vi "AODO-Configure AO.vi"(0 "AO.Channels":string[](array[string]), 5 "AO.Fs (Hz)":dbl, 7 "AO.Npts":i32, 11 "error in (no error)":errorcluster) -> (15 "error out":errorcluster)   [LabVIEW 2020]
uses:
  Typedefs/AODO-Action.ctl
  Typedefs/AODO-Config.ctl
  Typedefs/AODO-Output Spec.ctl
  Typedefs/DO-Output Spec.ctl
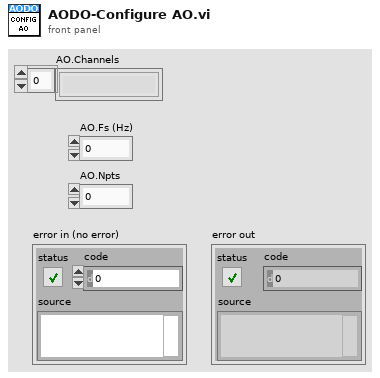
[diagram p1: front panel]
types:
  T1 = typedef "AODO-Config.ctl" = cluster{"AO":T2, "DO":T3, "hold outputs":bool, "ExtTrig":bool, "Trig Src":string}
  T2 = typedef "AODO-Output Spec.ctl" = cluster{"Channels":string[], "Fs (Hz)":dbl, "Npts":i32, "Gains":dbl[]}
  T3 = typedef "DO-Output Spec.ctl" = cluster{"Channels":string[], "Fs (Hz)":dbl, "Npts":i32, "Port":string}
  T4 = typedef "AODO-Action.ctl" = enum16{"Configure", "Initialize", "Start", "Write", "Clean up", "Init & Start", "Config & Test", "Position", "Set AO Gains", "Zero"}
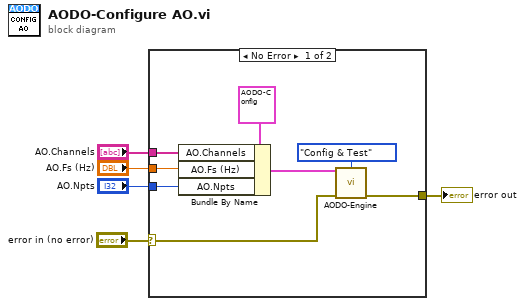
[diagram p0: block diagram]
diagram:
  n1 = case shown="No Error" "error in (no error)" {
    selector: "error in (no error)" -> [w7 w14]
    tunnel: "AO.Channels" -> [w10 _]
    tunnel: "AO.Fs (Hz)" -> [w9 _]
    tunnel: "AO.Npts" -> [w8 _]
    tunnel: [w6 w14] -> w1
    frame No Error {
      n2 = Bundle By Name(cluster=T1 {"AO"={"Channels"=[], "Fs (Hz)"=0.0, "Npts"=0, "Gains"=[]}, "DO"={"Channels"=[], "Fs (Hz)"=0.0, "Npts"=0, "Port"=""}, "hold outputs"=FALSE, "ExtTrig"=FALSE, "Trig Src"=""} ("Config"), "AO.Channels"=w10, "AO.Fs (Hz)"=w9, "AO.Npts"=w8) -> (w12:T1)
      n3 = call "AODO-Engine.vi"("Config"=w12, "Action"=AODO-Action."Config & Test", "error in (no error)"=w7) -> ("error out"=w6:errorcluster)  [unwired: 11 in, 1 out]
    }
    frame Error {
    }
  }
  "error out" <- w1
